vi "Self Initialization.vi"(8 "error in (no error)":errorcluster, 11 "Self Addressed Task in":refnum<class "Self Addressed Task.lvclass">) -> (0 "error out":errorcluster, 3 "Self Addressed Task out":refnum<class "Self Addressed Task.lvclass">)   [LabVIEW 2024, in "Self Addressed Task.lvclass"]
uses:
  Self Addressed Task.lvclass
  Self Addressed Task.lvclass/Self Addressed Task.ctl
  Task Ancestor/Task Ancestor.lvclass
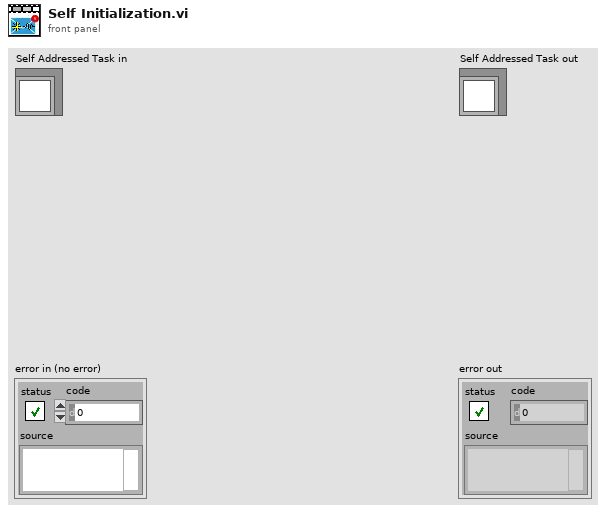
[diagram p1: front panel]
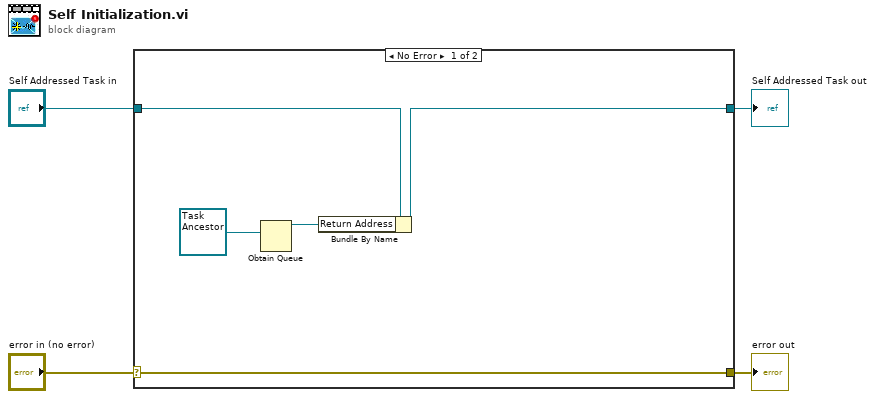
[diagram p0: block diagram]
diagram:
  n1 = case shown="No Error" "error in (no error)" {
    selector: "error in (no error)" -> [w9 w11]
    tunnel: [w9 w11] -> w3
    tunnel: [w5 w10] -> w1
    tunnel: "Self Addressed Task in" -> [w7 w10]
    frame No Error {
      n2 = Obtain Queue(element data type=refnum<class "Task Ancestor.lvclass"> refnum ("Task Ancestor.lvclass")) -> (queue out=w6:refnum<queue>)  [unwired: 4 in, 2 out]
      n3 = Bundle By Name(cluster=w7, "Return Address"=w6) -> (w5:refnum<class "Self Addressed Task.lvclass">)
    }
    frame Error {
    }
  }
  "error out" <- w3
  "Self Addressed Task out" <- w1
